vi "Right Button Pressed.vi"(8 "error in":errorcluster, 10 "variant":variant, 11 "ATM Data":T1={"UI Refs"={"Right Buttons"=refnum, "Left Buttons"=refnum, "User Input"=refnum, "ATM Messages"=refnum, "Left Menu"=refnum, "Right Menu"=refnum, "Enter"=refnum}, "Map"={}, "Login Valid?"=FALSE, "Queue Message"=refnum, "State"=enum."None", "User"={"Pin"="", "First Name"="", "Last Name"="", "Balance"=0.0, "Login Valid?"=FALSE}, "Main States"={"Message"="Initialize", "Data"=variant}}) -> (0 "error out":errorcluster, 3 "ATM Data Out":T1={"UI Refs"={"Right Buttons"=refnum, "Left Buttons"=refnum, "User Input"=refnum, "ATM Messages"=refnum, "Left Menu"=refnum, "Right Menu"=refnum, "Enter"=refnum}, "Map"={}, "Login Valid?"=FALSE, "Queue Message"=refnum, "State"=enum."None", "User"={"Pin"="", "First Name"="", "Last Name"="", "Balance"=0.0, "Login Valid?"=FALSE}, "Main States"={"Message"="Initialize", "Data"=variant}})   [LabVIEW 2020, in "ATM Machine.lvlib"]
uses:
  ATM Machine.lvlib
  Cluster - ATM Machine Data.ctl
  Cluster - Message Cluster.ctl
  Enum - ATM States.ctl
  98e35c26-2ff4-4b69-a813-136909b321a2.vi
  <vilib>/Comparison/Equal/Equal Functor/Equal Functor.lvclass
panel:
  out "element":string
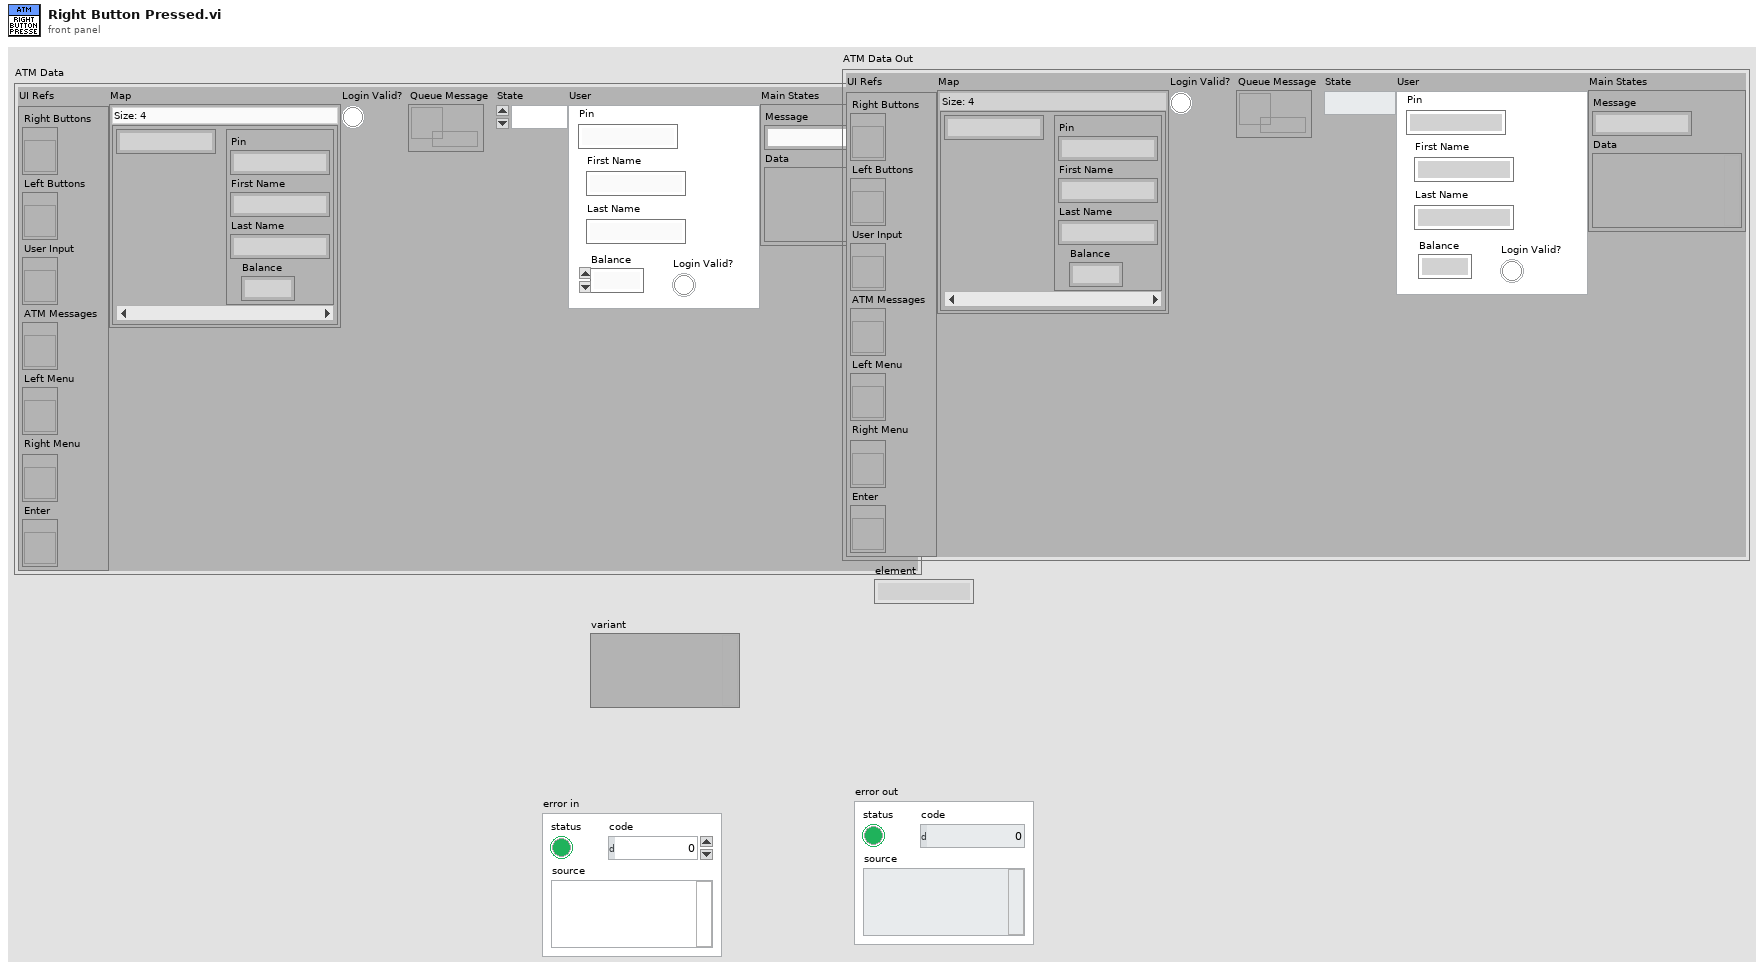
[diagram p1: front panel]
types:
  T1 = typedef "ATM Machine.lvlib/Cluster - ATM Machine Data.ctl" = cluster{"UI Refs":cluster{"Right Buttons":refnum<vi>, "Left Buttons":refnum<vi>, "User Input":refnum<vi>, "ATM Messages":refnum<vi>, "Left Menu":refnum<vi>, "Right Menu":refnum<vi>, "Enter":refnum<vi>}, "Map":map{string, cluster{"Pin":string, "First Name":string, "Last Name":string, "Balance":dbl}}, "Login Valid?":bool, "Queue Message":refnum<queue>, "State":T2, "User":cluster{"Pin":string, "First Name":string, "Last Name":string, "Balance":dbl, "Login Valid?":bool}, "Main States":cluster{"Message":string, "Data":variant}}
  T2 = typedef "ATM Machine.lvlib/Enum - ATM States.ctl" = enum16{"None", "Deposit", "Withdraw", "Card Inserted", "Balance Inquiry", "Return Card and Terminate", "Fast Cash"}
  T3 = cluster{"RFS String":string, "RFS String 2":string, "RFS String 3":string}
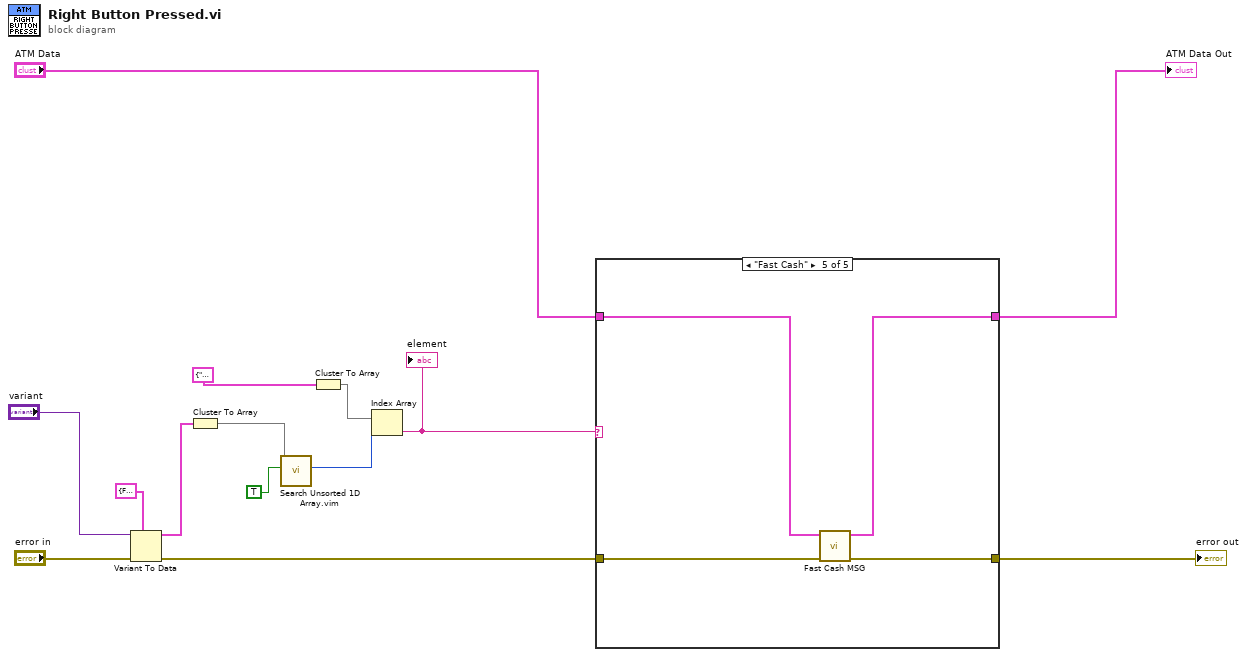
[diagram p0: block diagram]
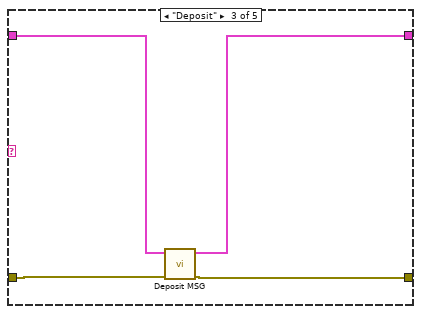
[diagram p4: hidden frame]
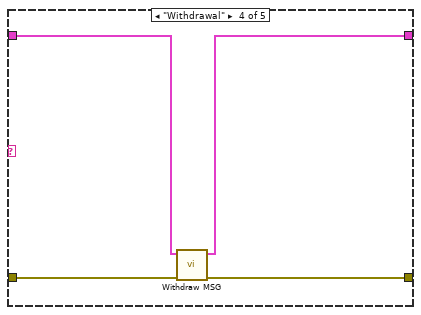
[diagram p5: hidden frame]
diagram:
  n1 = Variant To Data(error in="error in", type=cluster{bool, bool, bool} {FALSE, FALSE, FALSE}, Variant="variant") -> (data=w11:cluster{bool, bool, bool}, error out=w1:errorcluster)
  n2 = Cluster To Array(cluster=w11) -> (array=w10:bool[])
  n3 = call "Search Unsorted 1D Array.vim"("element"=TRUE, "unsorted 1D array"=w10) -> ("index of element"=w7:i32)  [unwired: 9 in]
  n4 = Cluster To Array(cluster=T3 {"RFS String"="Deposit", "RFS String 2"="Withdrawal", "RFS String 3"="Fast Cash"} ("Right Menu")) -> (array=w8:string[])
  n5 = Index Array(array=w8, index=w7) -> (element=w5:string)
  "element" <- w5
  n6 = case shown="\"Fast Cash\"" w5 {
    tunnel: "ATM Data" -> [w16 w18 w20 w26 w30]
    tunnel: [w16 w18 w19 w25 w29] -> w3
    tunnel: [w15 w17 w21 w23 w28] -> w2
    tunnel: w1 -> [w15 w17 w22 w24 w27]
    frame "False", Default {
    }
    frame "True" {
    }
    frame "Deposit" {
      n7 = call "Deposit MSG.vi"("error in"=w22, "ATM Data"=w20) -> ("error out"=w21:errorcluster, "ATM Data Out"=w19:T1)  [unwired: 8 in]
    }
    frame "Withdrawal" {
      n8 = call "Withdraw MSG.vi"("error in"=w24, "ATM Data"=w26) -> ("error out"=w23:errorcluster, "ATM Data Out"=w25:T1)  [unwired: 8 in]
    }
    frame "Fast Cash" {
      n9 = call "Fast Cash MSG.vi"("error in"=w27, "ATM Data"=w30) -> ("error out"=w28:errorcluster, "ATM Data Out"=w29:T1)  [unwired: 8 in]
    }
  }
  "ATM Data Out" <- w3
  "error out" <- w2
